vi "Set Listbox Item Symbol.vi"(6 "Row":i32, 7 "Listbox":refnum<vi>) -> (2 "dup Listboc":refnum<vi>)   [LabVIEW 2015]
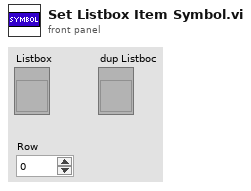
[diagram p1: front panel]
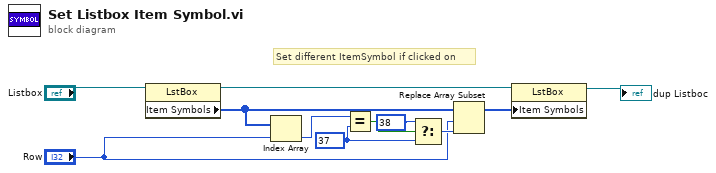
[diagram p0: block diagram]
diagram:
  w6 = 37
  # "Set different ItemSymbol if clicked on"
  n1 = property class="LstBox"(reference="Listbox") -> (reference out=w9:refnum<vi>, "Item Symbols"=w7:i32[])  [unwired: 1 in, 1 out]
  n2 = Index Array(array=w7, index="Row") -> (element=w4:i32)
  n3 = Equal?(x=w4, y=w6) -> (x = y?=w11:bool)
  n4 = Select(t=38, s=w11, f=w6) -> (s? t:f=w10:i32)
  n5 = Replace Array Subset(array=w7, new element=w10, index="Row") -> (w8:i32[])
  n6 = property class="LstBox"(reference=w9, "Item Symbols"=w8) -> (reference out=→"dup Listboc":refnum<vi>)  [unwired: 1 in, 1 out]
